vi "mess压力数据上传.vi"(0 "夹持力":dbl, 1 "Url":string="http://10.6.1.31:8080/MesInnerpackLineIO.asmx", 5 "压力":dbl, 7 "barcode":string="C0C50E0004010", 9 "wkc_no":string="SB-QN-304", 11 "error in (no error)":errorcluster caption="错误输入（无错误）") -> (4 "ValidateBarcode":string="True,10270194,C.0C.50E,Firehawk药物支架系统（CE无标签）RV3035,RV3035,10", 6 "数据上传OK/NG":bool, 15 "error out":errorcluster caption="错误输出")   [LabVIEW 2017]
uses:
  D:/Inspect System/Source Code/Andafa.IO.Helper.dll
  Andafa.IO.Helper.dll
panel:
  out "数组":string[](array[string])
  in  "wkc_time":timestamp
  in  "accessKey":string="a45b2d3334ffs_"
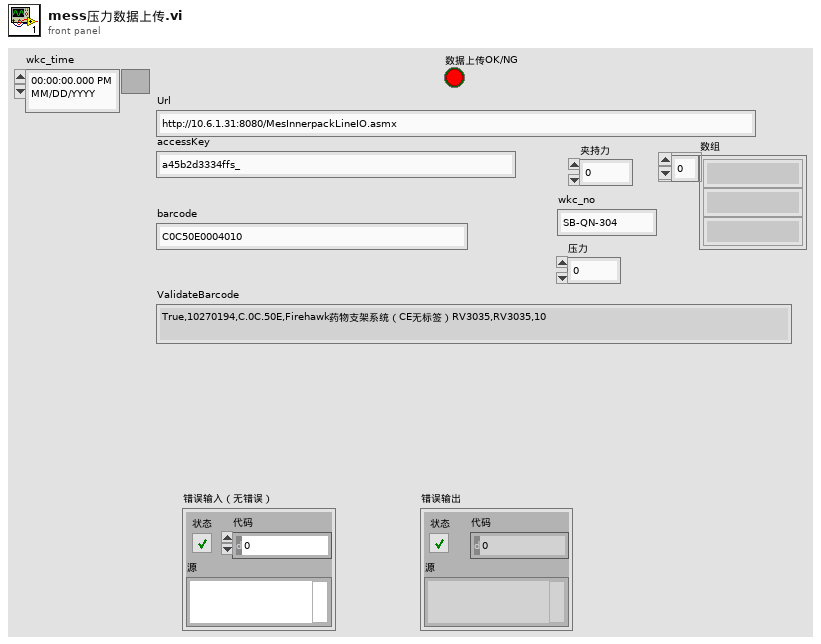
[diagram p1: front panel]
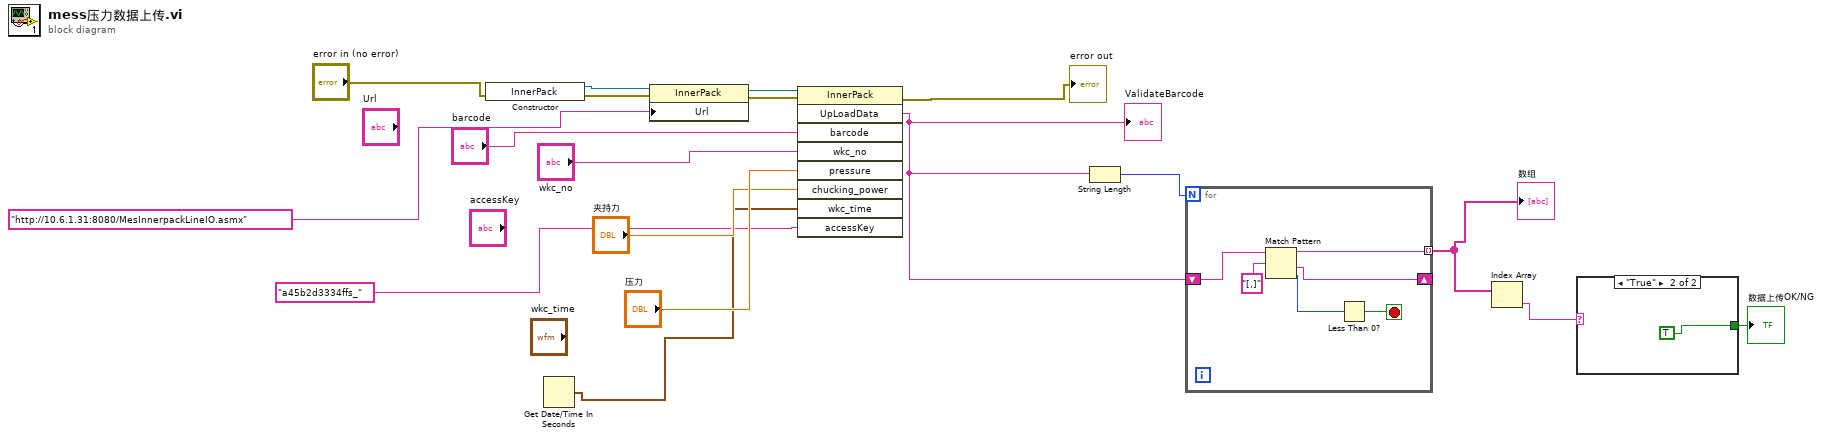
[diagram p0: block diagram]
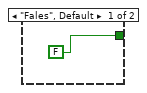
[diagram p2: hidden frame]
diagram:
  n1 = constructor class="InnerPack"(error in="error in (no error)") -> (reference out=w15:refnum<k24>, error out=w14:errorcluster)  [unwired: 2 in, 1 out]
  n2 = Get Date/Time In Seconds() -> (seconds since 1Jan1904=w5:timestamp)
  n3 = property on="属性节点" class="InnerPack"(reference=w15, error in=w14, "Url"="http://10.6.1.31:8080/MesInnerpackLineIO.asmx" ("accessKey")) -> (reference out=w13:refnum<k24>, error out=w12:errorcluster)
  n4 = invoke on="调用节点" class="InnerPack" method="UpLoadData"(reference=w13, error in=w12, "barcode"="barcode", "wkc_no"="wkc_no", "pressure"="压力", "chucking_power"="夹持力", "wkc_time"=w5, "accessKey"="a45b2d3334ffs_") -> (error out=→"error out":errorcluster, "UpLoadData"=w1:string)  [unwired: 1 in, 7 out]
  "ValidateBarcode" <- w1
  n5 = String Length(string=w1) -> (length=w2:i32)
  n6 = for {
    N: w2 -> [_]
    shift-right: [w21] -> _
    shift-left: w1 -> [w24]
    tunnel: [w22] -> w18 mode=indexing
    stop <- w19 stop-if-true
    n7 = Match Pattern(string=w24, regular expression="[,]" ("正则表达式")) -> (before substring=w22:string, after substring=w21:string, offset past match=w20:i32)  [unwired: 1 in, 1 out]
    n8 = Less Than 0?(x=w20) -> (x < 0?=w19:bool)
  }
  "数组" <- w18
  n9 = Index Array(array=w18) -> (element=w17:string)  [unwired: 1 in]
  n10 = case shown="\"True\"" w17 {
    tunnel: [FALSE TRUE] -> w16
    frame "Fales", Default {
    }
    frame "True" {
    }
  }
  "数据上传OK/NG" <- w16
